vi "Electrical_Data_IEEE1459.vi"(6 "Config":cluster{"k":i32, "f":i32, "fs":i32}, 7 "fase a":cluster{"va(t)":dbl[], "ia(t)":dbl[]}, 8 "fase c":cluster{"vc(t)":dbl[], "ic(t)":dbl[]}, 11 "fase b":cluster{"vb(t)":dbl[], "ib(t)":dbl[]}) -> (0 "FASE C":T2, 3 "FASE B":T3, 4 "TRIFASICO":T1, 5 "FASE A":T4)   [LabVIEW 2017]
uses:
  <vilib>/Analysis/2dsp.llb/Real FFT.vi
  <vilib>/Analysis/baseanly.llb/Mean (DBL).vi
  <vilib>/Analysis/NI_AALPro.lvlib
  <vilib>/Analysis/NI_AALBase.lvlib
panel:
  in  "Cfg3F":T1
  in  "CfgC":T2
  in  "CfgB":T3
  in  "CfgA":T4
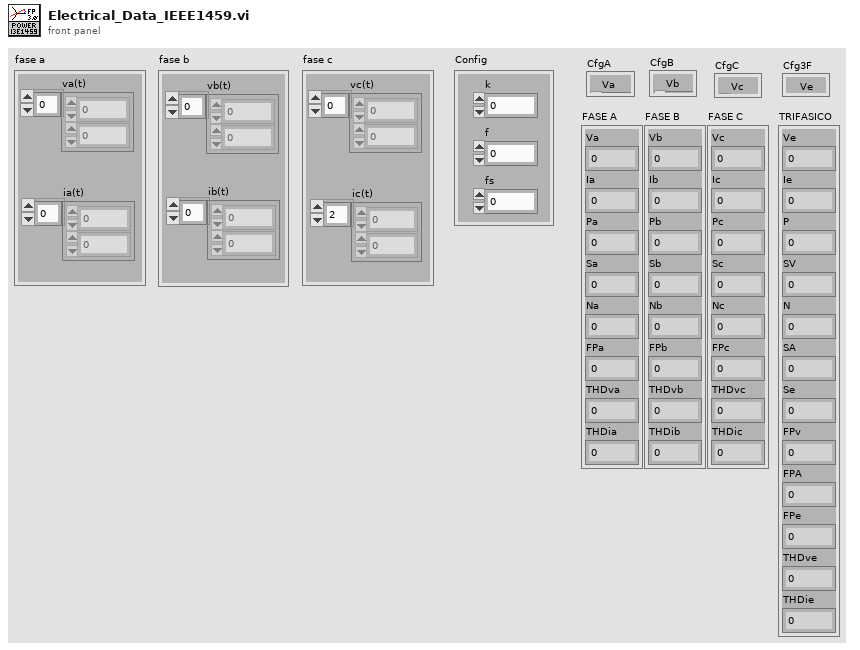
[diagram p1: front panel]
types:
  T1 = cluster{"Ve":dbl, "Ie":dbl, "P":dbl, "SV":dbl, "N":dbl, "SA":dbl, "Se":dbl, "FPv":dbl, "FPA":dbl, "FPe":dbl, "THDve":dbl, "THDie":dbl}
  T2 = cluster{"Vc":dbl, "Ic":dbl, "Pc":dbl, "Sc":dbl, "Nc":dbl, "FPc":dbl, "THDvc":dbl, "THDic":dbl}
  T3 = cluster{"Vb":dbl, "Ib":dbl, "Pb":dbl, "Sb":dbl, "Nb":dbl, "FPb":dbl, "THDvb":dbl, "THDib":dbl}
  T4 = cluster{"Va":dbl, "Ia":dbl, "Pa":dbl, "Sa":dbl, "Na":dbl, "FPa":dbl, "THDva":dbl, "THDia":dbl}
  T5 = cluster{cdb[], cdb[], cdb[], cdb[], cdb[], cdb[], cdb[], cdb[], cdb[], cdb[]}
  T6 = cluster{cdb[], cdb[], cdb[], cdb[], cdb[], cdb[]}
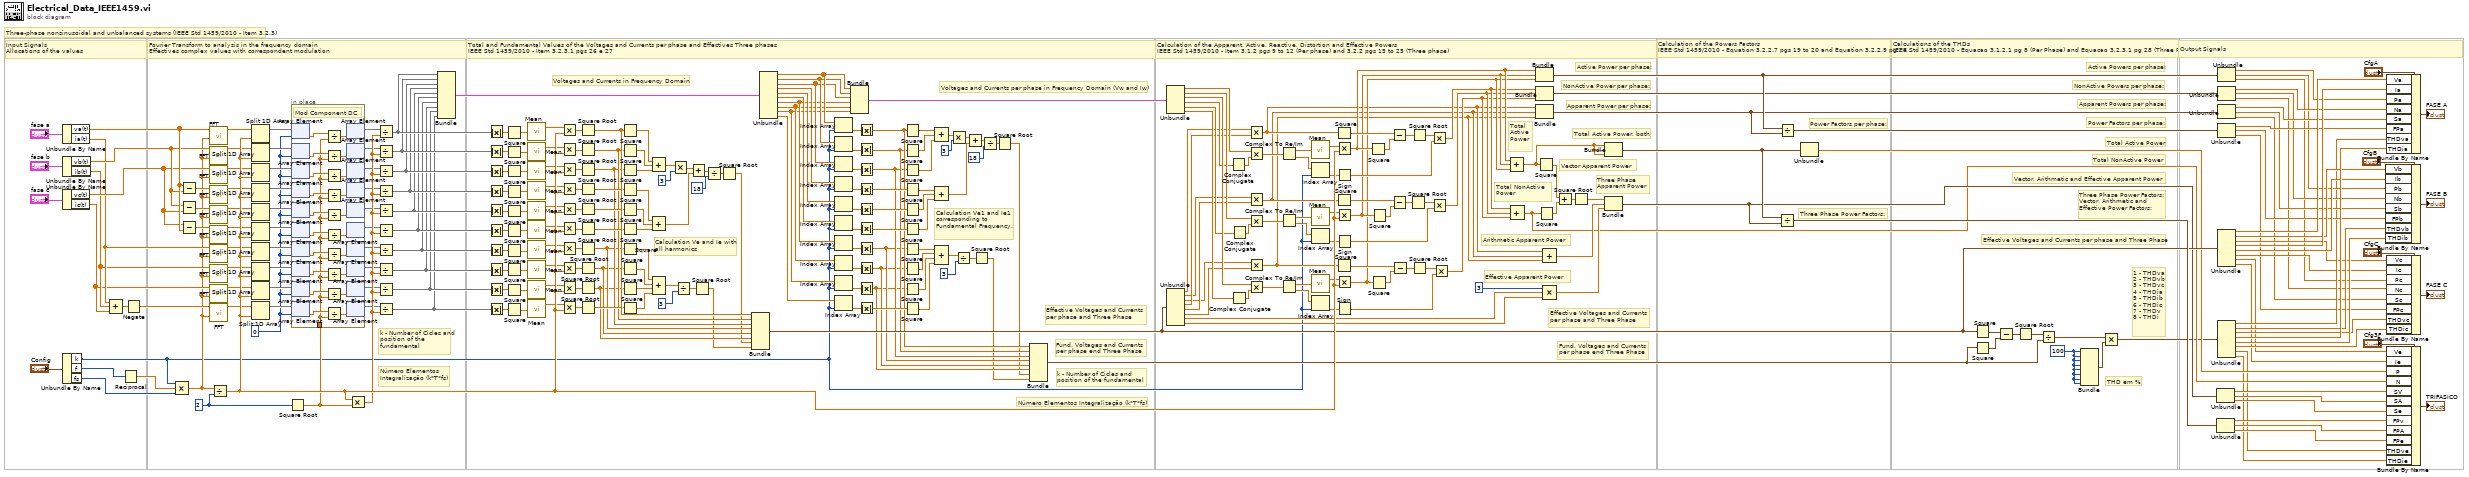
[diagram p0: block diagram]
diagram:
  w2 = i8 100
  w247 = 0 ("index")
  w268 = i8 2 ("y")
  # "THD em %"
  # "Three Phase Power Factors:"
  # "Power Factors per phase:"
  # "Vector, Arithmetic and Effective Apparent Power"
  # "Total Active Power"
  # "Active Powers per phase:"
  # "NonActive Powers per phase:"
  # "Apparent Powers per phase:"
  # "Total NonActive Power"
  # "Power Factors per phase:"
  # "Three Phase Power Factors:\nVector, Arithmetic and Effective Power Factors:"
  # "Effective Voltages and Currents per phase and Three Phase"
  # "1 - THDva\n2 - THDvb\n3 - THDvc\n4 - THDia\n5 - THDib\n6 - THDic\n7 - THDv\n8 - THDi"
  # "Three Phase Apparent Power"
  # "Total Active Power, both"
  # "Apparent Power per phase:"
  # "NonActive Power per phase:"
  # "Active Power per phase:"
  # "Effective Voltages and Currents per phase and Three Phase"
  # "Fund. Voltages and Currents per phase end Three Phase"
  # "Vector Apparent Power"
  # "Total NonActive Power"
  # "Total Active Power"
  # "Effective Apparent Power"
  # "Arithmetic Apparent Power"
  # "Voltages and Currents in Frequency Domain"
  # "Voltages and Currents per phase in Frequency Domain (Vw and Iw)"
  # "Fund. Voltages and Currents per phase end Three Phase"
  # "Effective Voltages and Currents per phase and Three Phase"
  # "Número Elementos Integralização (k*T*fs)"
  # "k - Number of Cicles and position of the fundamental"
  # "Calculation Ve1 and Ie1 corresponding to Fundamental Frequency."
  # "Calculation Ve and Ie with\nall harmonics"
  # "k - Number of Cicles and position of the fundamental"
  # "Número Elementos Integralização (k*T*fs)"
  # "Three-phase nonsinusoidal and unbalanced systems (IEEE Std 1459/2010 - Ítem 3.2.3)"
  # "Input Signals\nAllocations of the values"
  # "Output Signals"
  # "Calculations of the THDs\nIEEE Std 1459/2010 - Equacao 3.1.2.1 pg 8 (Per Phase) and Equacao 3.2.3.1 pg 28 (Three Phase)"
  # "Calculation of the Powers Factors\nIEEE Std 1459/2010 - Equation 3.2.2.7 pgs 19 to 20 and Equation 3.2.2.9 pg 24"
  # "Calculation of the Apparent, Active, Reactive, Distortion and Effective Powers\nIEEE Std 1459/2010 - Ítem 3.1.2 pgs 9 to 12 (Per phase) and 3.2.2 pgs 15 to 25 (Three phase)"
  # "Total and Fundamental Values of the Voltages and Currents per phase and Effectives Three phases\nIEEE Std 1459/2010 - Ítem 3.2.3.1 pgs 26 e 27"
  # "Fourier Transform to analysis in the frequency domain\nEffectives complex values with correspondent modulation"
  n1 = Unbundle By Name("fase a") -> ("va(t)"=w305:dbl[], "ia(t)"=w300:dbl[])
  n2 = Unbundle By Name("fase b") -> ("vb(t)"=w304:dbl[], "ib(t)"=w299:dbl[])
  n3 = Unbundle By Name("fase c") -> ("vc(t)"=w303:dbl[], "ic(t)"=w298:dbl[])
  n4 = Unbundle By Name("Config") -> ("k"=w15:i32, "f"=w13:i32, "fs"=w14:i32)
  n5 = Compound Arithmetic op=ADD(w300, w299, w298) -> (w287:dbl[])
  n6 = Reciprocal(x=w13) -> (1/x=w302:dbl)
  n7 = Negate(x=w287) -> (-x=w301:dbl[])
  n8 = Compound Arithmetic op=MULTIPLY(w15, w302, w14) -> (w280:dbl)
  n9 = Subtract(x=w305, y=w304) -> (x-y=w283:dbl[])
  n10 = Subtract(x=w304, y=w303) -> (x-y=w282:dbl[])
  n11 = Subtract(x=w303, y=w305) -> (x-y=w281:dbl[])
  n12 = call-poly <vilib>:"FFT.vi"("FFT size"=w280, "X"=w305) -> ("FFT {X}"=w279:cdb[])  [unwired: 8 in, 1 out]
  n13 = call-poly <vilib>:"FFT.vi"("FFT size"=w280, "X"=w304) -> ("FFT {X}"=w277:cdb[])  [unwired: 8 in, 1 out]
  n14 = call-poly <vilib>:"FFT.vi"("FFT size"=w280, "X"=w303) -> ("FFT {X}"=w276:cdb[])  [unwired: 8 in, 1 out]
  n15 = call-poly <vilib>:"FFT.vi"("FFT size"=w280, "X"=w283) -> ("FFT {X}"=w275:cdb[])  [unwired: 8 in, 1 out]
  n16 = call-poly <vilib>:"FFT.vi"("FFT size"=w280, "X"=w282) -> ("FFT {X}"=w274:cdb[])  [unwired: 8 in, 1 out]
  n17 = call-poly <vilib>:"FFT.vi"("FFT size"=w280, "X"=w281) -> ("FFT {X}"=w273:cdb[])  [unwired: 8 in, 1 out]
  n18 = call-poly <vilib>:"FFT.vi"("FFT size"=w280, "X"=w300) -> ("FFT {X}"=w272:cdb[])  [unwired: 8 in, 1 out]
  n19 = call-poly <vilib>:"FFT.vi"("FFT size"=w280, "X"=w299) -> ("FFT {X}"=w271:cdb[])  [unwired: 8 in, 1 out]
  n20 = call-poly <vilib>:"FFT.vi"("FFT size"=w280, "X"=w298) -> ("FFT {X}"=w270:cdb[])  [unwired: 8 in, 1 out]
  n21 = call-poly <vilib>:"FFT.vi"("FFT size"=w280, "X"=w301) -> ("FFT {X}"=w278:cdb[])  [unwired: 8 in, 1 out]
  n22 = Divide(x=w280, y=w268) -> (x/y=w306:dbl)
  n23 = Split 1D Array(array=w279, index=w306) -> (first subarray=w267:cdb[])  [unwired: 1 out]
  n24 = Split 1D Array(array=w277, index=w306) -> (first subarray=w266:cdb[])  [unwired: 1 out]
  n25 = Split 1D Array(array=w276, index=w306) -> (first subarray=w265:cdb[])  [unwired: 1 out]
  n26 = Split 1D Array(array=w275, index=w306) -> (first subarray=w264:cdb[])  [unwired: 1 out]
  n27 = Split 1D Array(array=w274, index=w306) -> (first subarray=w263:cdb[])  [unwired: 1 out]
  n28 = Split 1D Array(array=w273, index=w306) -> (first subarray=w262:cdb[])  [unwired: 1 out]
  n29 = Split 1D Array(array=w272, index=w306) -> (first subarray=w261:cdb[])  [unwired: 1 out]
  n30 = Split 1D Array(array=w271, index=w306) -> (first subarray=w260:cdb[])  [unwired: 1 out]
  n31 = Split 1D Array(array=w270, index=w306) -> (first subarray=w259:cdb[])  [unwired: 1 out]
  n32 = Split 1D Array(array=w278, index=w306) -> (first subarray=w258:cdb[])  [unwired: 1 out]
  n33 = Square Root(x=w268) -> (sqrt(x)=w246:dbl)
  n34 = in-place {
    in-place-border: w246 -> [w317]
    # "Mod Component DC"
    n35 = in-place-array #1(w267, w247) -> (w318:cdb)
    n36 = in-place-array #2(w266, w247) -> (w319:cdb)
    n37 = in-place-array #3(w265, w247) -> (w320:cdb)
    n38 = in-place-array #4(w264, w247) -> (w321:cdb)
    n39 = in-place-array #5(w263, w247) -> (w322:cdb)
    n40 = in-place-array #6(w262, w247) -> (w323:cdb)
    n41 = in-place-array #7(w261, w247) -> (w324:cdb)
    n42 = in-place-array #8(w260, w247) -> (w325:cdb)
    n43 = in-place-array #9(w259, w247) -> (w326:cdb)
    n44 = in-place-array #10(w258, w247) -> (w327:cdb)
    n45 = Divide(x=w318, y=w317) -> (x/y=w336:cdb)
    n46 = Divide(x=w319, y=w317) -> (x/y=w328:cdb)
    n47 = Divide(x=w320, y=w317) -> (x/y=w329:cdb)
    n48 = Divide(x=w321, y=w317) -> (x/y=w330:cdb)
    n49 = Divide(x=w322, y=w317) -> (x/y=w331:cdb)
    n50 = Divide(x=w323, y=w317) -> (x/y=w332:cdb)
    n51 = Divide(x=w324, y=w317) -> (x/y=w333:cdb)
    n52 = Divide(x=w325, y=w317) -> (x/y=w334:cdb)
    n53 = Divide(x=w326, y=w317) -> (x/y=w335:cdb)
    n54 = Divide(x=w327, y=w317) -> (x/y=w337:cdb)
    n55 = in-place-array #1(w336) -> (w255:cdb[])  [unwired: 1 out]
    n56 = in-place-array #2(w328) -> (w256:cdb[])  [unwired: 1 out]
    n57 = in-place-array #3(w329) -> (w257:cdb[])  [unwired: 1 out]
    n58 = in-place-array #4(w330) -> (w254:cdb[])  [unwired: 1 out]
    n59 = in-place-array #5(w331) -> (w253:cdb[])  [unwired: 1 out]
    n60 = in-place-array #6(w332) -> (w252:cdb[])  [unwired: 1 out]
    n61 = in-place-array #7(w333) -> (w251:cdb[])  [unwired: 1 out]
    n62 = in-place-array #8(w334) -> (w250:cdb[])  [unwired: 1 out]
    n63 = in-place-array #9(w335) -> (w249:cdb[])  [unwired: 1 out]
    n64 = in-place-array #10(w337) -> (w248:cdb[])  [unwired: 1 out]
  }
  n65 = Multiply(x=w306, y=w246) -> (x*y=w269:dbl)
  n66 = Divide(x=w255, y=w269) -> (x/y=w316:cdb[])
  n67 = Divide(x=w256, y=w269) -> (x/y=w315:cdb[])
  n68 = Divide(x=w257, y=w269) -> (x/y=w314:cdb[])
  n69 = Divide(x=w254, y=w269) -> (x/y=w313:cdb[])
  n70 = Divide(x=w253, y=w269) -> (x/y=w312:cdb[])
  n71 = Divide(x=w252, y=w269) -> (x/y=w311:cdb[])
  n72 = Divide(x=w251, y=w269) -> (x/y=w310:cdb[])
  n73 = Divide(x=w250, y=w269) -> (x/y=w309:cdb[])
  n74 = Divide(x=w249, y=w269) -> (x/y=w308:cdb[])
  n75 = Divide(x=w248, y=w269) -> (x/y=w307:cdb[])
  n76 = Bundle(w316, w315, w314, w313, w312, w311, w310, w309, w308, w307) -> (w297:T5)  [unwired: 1 in]
  n77 = Absolute Value(x=w316) -> (abs(x)=w245:dbl[])
  n78 = Absolute Value(x=w315) -> (abs(x)=w244:dbl[])
  n79 = Absolute Value(x=w314) -> (abs(x)=w243:dbl[])
  n80 = Absolute Value(x=w313) -> (abs(x)=w168:dbl[])
  n81 = Absolute Value(x=w312) -> (abs(x)=w242:dbl[])
  n82 = Absolute Value(x=w311) -> (abs(x)=w241:dbl[])
  n83 = Absolute Value(x=w310) -> (abs(x)=w240:dbl[])
  n84 = Absolute Value(x=w309) -> (abs(x)=w239:dbl[])
  n85 = Absolute Value(x=w308) -> (abs(x)=w238:dbl[])
  n86 = Absolute Value(x=w307) -> (abs(x)=w237:dbl[])
  n87 = Square(x=w245) -> (x^2=w227:dbl[])
  n88 = Square(x=w244) -> (x^2=w228:dbl[])
  n89 = Square(x=w243) -> (x^2=w229:dbl[])
  n90 = Square(x=w168) -> (x^2=w230:dbl[])
  n91 = Square(x=w242) -> (x^2=w231:dbl[])
  n92 = Square(x=w241) -> (x^2=w232:dbl[])
  n93 = Square(x=w240) -> (x^2=w233:dbl[])
  n94 = Square(x=w239) -> (x^2=w234:dbl[])
  n95 = Square(x=w238) -> (x^2=w235:dbl[])
  n96 = Square(x=w237) -> (x^2=w236:dbl[])
  n97 = call-poly <vilib>:"Mean.vi"("X"=w227) -> ("mean"=w226:dbl)  [unwired: 1 out]
  n98 = call-poly <vilib>:"Mean.vi"("X"=w228) -> ("mean"=w207:dbl)  [unwired: 1 out]
  n99 = call-poly <vilib>:"Mean.vi"("X"=w229) -> ("mean"=w208:dbl)  [unwired: 1 out]
  n100 = call-poly <vilib>:"Mean.vi"("X"=w230) -> ("mean"=w209:dbl)  [unwired: 1 out]
  n101 = call-poly <vilib>:"Mean.vi"("X"=w231) -> ("mean"=w210:dbl)  [unwired: 1 out]
  n102 = call-poly <vilib>:"Mean.vi"("X"=w232) -> ("mean"=w211:dbl)  [unwired: 1 out]
  n103 = call-poly <vilib>:"Mean.vi"("X"=w233) -> ("mean"=w212:dbl)  [unwired: 1 out]
  n104 = call-poly <vilib>:"Mean.vi"("X"=w234) -> ("mean"=w213:dbl)  [unwired: 1 out]
  n105 = call-poly <vilib>:"Mean.vi"("X"=w235) -> ("mean"=w214:dbl)  [unwired: 1 out]
  n106 = call-poly <vilib>:"Mean.vi"("X"=w236) -> ("mean"=w224:dbl)  [unwired: 1 out]
  n107 = Multiply(x=w226, y=w306) -> (x*y=w225:dbl)
  n108 = Multiply(x=w207, y=w306) -> (x*y=w222:dbl)
  n109 = Multiply(x=w208, y=w306) -> (x*y=w221:dbl)
  n110 = Multiply(x=w209, y=w306) -> (x*y=w220:dbl)
  n111 = Multiply(x=w210, y=w306) -> (x*y=w219:dbl)
  n112 = Multiply(x=w211, y=w306) -> (x*y=w218:dbl)
  n113 = Multiply(x=w212, y=w306) -> (x*y=w217:dbl)
  n114 = Multiply(x=w213, y=w306) -> (x*y=w216:dbl)
  n115 = Multiply(x=w214, y=w306) -> (x*y=w215:dbl)
  n116 = Multiply(x=w224, y=w306) -> (x*y=w223:dbl)
  n117 = Square Root(x=w225) -> (sqrt(x)=w147:dbl)
  n118 = Square Root(x=w222) -> (sqrt(x)=w128:dbl)
  n119 = Square Root(x=w221) -> (sqrt(x)=w127:dbl)
  n120 = Square Root(x=w220) -> (sqrt(x)=w146:dbl)
  n121 = Square Root(x=w219) -> (sqrt(x)=w145:dbl)
  n122 = Square Root(x=w218) -> (sqrt(x)=w144:dbl)
  n123 = Square Root(x=w217) -> (sqrt(x)=w126:dbl)
  n124 = Square Root(x=w216) -> (sqrt(x)=w125:dbl)
  n125 = Square Root(x=w215) -> (sqrt(x)=w124:dbl)
  n126 = Square Root(x=w223) -> (sqrt(x)=w143:dbl)
  n127 = Square(x=w147) -> (x^2=w200:dbl)
  n128 = Square(x=w128) -> (x^2=w199:dbl)
  n129 = Square(x=w127) -> (x^2=w198:dbl)
  n130 = Square(x=w146) -> (x^2=w197:dbl)
  n131 = Square(x=w145) -> (x^2=w196:dbl)
  n132 = Square(x=w144) -> (x^2=w195:dbl)
  n133 = Square(x=w126) -> (x^2=w205:dbl)
  n134 = Square(x=w125) -> (x^2=w204:dbl)
  n135 = Square(x=w124) -> (x^2=w203:dbl)
  n136 = Square(x=w143) -> (x^2=w202:dbl)
  n137 = Compound Arithmetic op=ADD(w200, w199, w198) -> (w194:dbl)
  n138 = Compound Arithmetic op=ADD(w197, w196, w195) -> (w192:dbl)
  n139 = Compound Arithmetic op=ADD(w205, w204, w203, w202) -> (w201:dbl)
  n140 = Multiply(x=w194, y=i8 3) -> (x*y=w193:dbl)
  n141 = Divide(x=w201, y=i8 3) -> (x/y=w206:dbl)
  n142 = Add(x=w193, y=w192) -> (x+y=w190:dbl)
  n143 = Square Root(x=w206) -> (sqrt(x)=w123:dbl)
  n144 = Divide(x=w190, y=i8 18) -> (x/y=w191:dbl)
  n145 = Square Root(x=w191) -> (sqrt(x)=w122:dbl)
  n146 = Bundle(w147, w128, w127, w126, w125, w124, w122, w123) -> (w288:cluster{dbl, dbl, dbl, dbl, dbl, dbl, dbl, dbl})  [unwired: 1 in]
  n147 = Unbundle(w297) -> (w134:cdb[], w133:cdb[], w132:cdb[], w151:cdb[], w150:cdb[], w149:cdb[], w131:cdb[], w130:cdb[], w129:cdb[], w148:cdb[])
  n148 = Index Array(array=w134, index=w15) -> (element=w154:cdb)
  n149 = Index Array(array=w133, index=w15) -> (element=w155:cdb)
  n150 = Index Array(array=w132, index=w15) -> (element=w156:cdb)
  n151 = Index Array(array=w151, index=w15) -> (element=w157:cdb)
  n152 = Index Array(array=w150, index=w15) -> (element=w160:cdb)
  n153 = Index Array(array=w149, index=w15) -> (element=w161:cdb)
  n154 = Index Array(array=w131, index=w15) -> (element=w163:cdb)
  n155 = Index Array(array=w130, index=w15) -> (element=w164:cdb)
  n156 = Index Array(array=w129, index=w15) -> (element=w165:cdb)
  n157 = Index Array(array=w148, index=w15) -> (element=w166:cdb)
  n158 = Bundle(w134, w133, w132, w131, w130, w129) -> (w296:T6)  [unwired: 1 in]
  n159 = Absolute Value(x=w154) -> (abs(x)=w142:dbl)
  n160 = Absolute Value(x=w155) -> (abs(x)=w141:dbl)
  n161 = Absolute Value(x=w156) -> (abs(x)=w140:dbl)
  n162 = Absolute Value(x=w157) -> (abs(x)=w158:dbl)
  n163 = Absolute Value(x=w160) -> (abs(x)=w159:dbl)
  n164 = Absolute Value(x=w161) -> (abs(x)=w162:dbl)
  n165 = Absolute Value(x=w163) -> (abs(x)=w139:dbl)
  n166 = Absolute Value(x=w164) -> (abs(x)=w138:dbl)
  n167 = Absolute Value(x=w165) -> (abs(x)=w137:dbl)
  n168 = Absolute Value(x=w166) -> (abs(x)=w167:dbl)
  n169 = Square(x=w142) -> (x^2=w174:dbl)
  n170 = Square(x=w141) -> (x^2=w175:dbl)
  n171 = Square(x=w140) -> (x^2=w153:dbl)
  n172 = Square(x=w158) -> (x^2=w176:dbl)
  n173 = Square(x=w159) -> (x^2=w177:dbl)
  n174 = Square(x=w162) -> (x^2=w178:dbl)
  n175 = Square(x=w139) -> (x^2=w170:dbl)
  n176 = Square(x=w138) -> (x^2=w171:dbl)
  n177 = Square(x=w137) -> (x^2=w152:dbl)
  n178 = Square(x=w167) -> (x^2=w172:dbl)
  n179 = Compound Arithmetic op=ADD(w174, w175, w153) -> (w179:dbl)
  n180 = Compound Arithmetic op=ADD(w176, w177, w178) -> (w181:dbl)
  n181 = Compound Arithmetic op=ADD(w170, w171, w152, w172) -> (w173:dbl)
  n182 = Multiply(x=w179, y=i8 3) -> (x*y=w180:dbl)
  n183 = Divide(x=w173, y=i8 3) -> (x/y=w169:dbl)
  n184 = Add(x=w180, y=w181) -> (x+y=w183:dbl)
  n185 = Square Root(x=w169) -> (sqrt(x)=w135:dbl)
  n186 = Divide(x=w183, y=i8 18) -> (x/y=w182:dbl)
  n187 = Square Root(x=w182) -> (sqrt(x)=w136:dbl)
  n188 = Bundle(w142, w141, w140, w139, w138, w137, w136, w135) -> (w294:cluster{dbl, dbl, dbl, dbl, dbl, dbl, dbl, dbl})  [unwired: 1 in]
  n189 = Unbundle(w296) -> (w84:cdb[], w83:cdb[], w82:cdb[], w81:cdb[], w80:cdb[], w79:cdb[])
  n190 = Unbundle(w288) -> (w59:dbl, w57:dbl, w55:dbl, w58:dbl, w56:dbl, w54:dbl, w78:dbl, w77:dbl)
  n191 = Complex Conjugate(1:w81) -> (0:w119:cdb[])
  n192 = Complex Conjugate(1:w79) -> (0:w121:cdb[])
  n193 = Complex Conjugate(1:w80) -> (0:w120:cdb[])
  n194 = Multiply(x=w59, y=w58) -> (x*y=w70:dbl)
  n195 = Multiply(x=w84, y=w119) -> (x*y=w118:cdb[])
  n196 = Multiply(x=w57, y=w56) -> (x*y=w69:dbl)
  n197 = Multiply(x=w83, y=w120) -> (x*y=w117:cdb[])
  n198 = Multiply(x=w55, y=w54) -> (x*y=w68:dbl)
  n199 = Multiply(x=w82, y=w121) -> (x*y=w116:cdb[])
  n200 = Complex To Re/Im(x + iy=w118) -> (x=w115:dbl[], y=w105:dbl[])
  n201 = Complex To Re/Im(x + iy=w117) -> (x=w114:dbl[], y=w104:dbl[])
  n202 = Complex To Re/Im(x + iy=w116) -> (x=w113:dbl[], y=w103:dbl[])
  n203 = call-poly <vilib>:"Mean.vi"("X"=w115) -> ("mean"=w112:dbl)  [unwired: 1 out]
  n204 = Index Array(array=w105, index=w15) -> (element=w95:dbl)
  n205 = call-poly <vilib>:"Mean.vi"("X"=w114) -> ("mean"=w110:dbl)  [unwired: 1 out]
  n206 = Index Array(array=w104, index=w15) -> (element=w96:dbl)
  n207 = call-poly <vilib>:"Mean.vi"("X"=w113) -> ("mean"=w111:dbl)  [unwired: 1 out]
  n208 = Index Array(array=w103, index=w15) -> (element=w97:dbl)
  n209 = Square(x=w70) -> (x^2=w101:dbl)
  n210 = Square(x=w69) -> (x^2=w98:dbl)
  n211 = Square(x=w68) -> (x^2=w91:dbl)
  n212 = Multiply(x=w112, y=w306) -> (x*y=w76:dbl)
  n213 = Sign(1:w95) -> (0:w94:dbl)
  n214 = Multiply(x=w110, y=w306) -> (x*y=w75:dbl)
  n215 = Sign(1:w96) -> (0:w93:dbl)
  n216 = Multiply(x=w111, y=w306) -> (x*y=w74:dbl)
  n217 = Sign(1:w97) -> (0:w92:dbl)
  n218 = Square(x=w76) -> (x^2=w102:dbl)
  n219 = Square(x=w74) -> (x^2=w99:dbl)
  n220 = Square(x=w75) -> (x^2=w100:dbl)
  n221 = Subtract(x=w101, y=w102) -> (x-y=w90:dbl)
  n222 = Subtract(x=w98, y=w100) -> (x-y=w88:dbl)
  n223 = Subtract(x=w91, y=w99) -> (x-y=w86:dbl)
  n224 = Square Root(x=w88) -> (sqrt(x)=w87:dbl)
  n225 = Square Root(x=w90) -> (sqrt(x)=w89:dbl)
  n226 = Square Root(x=w86) -> (sqrt(x)=w85:dbl)
  n227 = Multiply(x=w89, y=w94) -> (x*y=w73:dbl)
  n228 = Multiply(x=w87, y=w93) -> (x*y=w72:dbl)
  n229 = Multiply(x=w85, y=w92) -> (x*y=w71:dbl)
  n230 = Compound Arithmetic op=ADD(w76, w75, w74) -> (w64:dbl)
  n231 = Compound Arithmetic op=ADD(w73, w72, w71) -> (w23:dbl)
  n232 = Bundle(w76, w75, w74) -> (w293:cluster{dbl, dbl, dbl})  [unwired: 1 in]
  n233 = Bundle(w73, w72, w71) -> (w292:cluster{dbl, dbl, dbl})  [unwired: 1 in]
  n234 = Bundle(w70, w69, w68) -> (w291:cluster{dbl, dbl, dbl})  [unwired: 1 in]
  n235 = Square(x=w64) -> (x^2=w107:dbl)
  n236 = Square(x=w23) -> (x^2=w106:dbl)
  n237 = Compound Arithmetic op=ADD(w70, w69, w68) -> (w66:dbl)
  n238 = Compound Arithmetic op=MULTIPLY(i8 3 ("value"), w78, w77) -> (w67:dbl)
  n239 = Add(x=w107, y=w106) -> (x+y=w108:dbl)
  n240 = Square Root(x=w108) -> (sqrt(x)=w65:dbl)
  n241 = Bundle(w65, w66, w67) -> (w25:cluster{dbl, dbl, dbl})  [unwired: 1 in]
  n242 = Bundle(w64, w64, w64) -> (w295:cluster{dbl, dbl, dbl})  [unwired: 1 in]
  n243 = Divide(x=w295, y=w25) -> (x/y=w289:cluster{dbl, dbl, dbl})
  n244 = Divide(x=w293, y=w291) -> (x/y=w290:cluster{dbl, dbl, dbl})
  n245 = Unbundle(w295) -> (w24:dbl)  [unwired: 2 out]
  n246 = Square(x=w288) -> (x^2=w63:cluster{dbl, dbl, dbl, dbl, dbl, dbl, dbl, dbl})
  n247 = Square(x=w294) -> (x^2=w62:cluster{dbl, dbl, dbl, dbl, dbl, dbl, dbl, dbl})
  n248 = Subtract(x=w63, y=w62) -> (x-y=w60:cluster{dbl, dbl, dbl, dbl, dbl, dbl, dbl, dbl})
  n249 = Square Root(x=w60) -> (sqrt(x)=w61:cluster{dbl, dbl, dbl, dbl, dbl, dbl, dbl, dbl})
  n250 = Divide(x=w61, y=w294) -> (x/y=w4:cluster{dbl, dbl, dbl, dbl, dbl, dbl, dbl, dbl})
  n251 = Bundle(w2, w2, w2, w2, w2, w2, w2, w2) -> (w1:cluster{i8, i8, i8, i8, i8, i8, i8, i8})  [unwired: 1 in]
  n252 = Multiply(x=w4, y=w1) -> (x*y=w3:cluster{dbl, dbl, dbl, dbl, dbl, dbl, dbl, dbl})
  n253 = Unbundle(w25) -> (w22:dbl, w21:dbl, w20:dbl)
  n254 = Unbundle(w289) -> (w19:dbl, w18:dbl, w17:dbl)
  n255 = Unbundle(w293) -> (w50:dbl, w42:dbl, w32:dbl)
  n256 = Unbundle(w292) -> (w49:dbl, w41:dbl, w31:dbl)
  n257 = Unbundle(w291) -> (w48:dbl, w40:dbl, w30:dbl)
  n258 = Unbundle(w290) -> (w46:dbl, w39:dbl, w29:dbl)
  n259 = Unbundle(w288) -> (w52:dbl, w44:dbl, w34:dbl, w51:dbl, w43:dbl, w33:dbl, w12:dbl, w11:dbl)
  n260 = Unbundle(w3) -> (w36:dbl, w38:dbl, w28:dbl, w47:dbl, w37:dbl, w26:dbl, w10:dbl, w9:dbl)
  n261 = Bundle By Name(cluster="CfgB", "Vb"=w44, "Ib"=w43, "Pb"=w42, "Nb"=w41, "Sb"=w40, "FPb"=w39, "THDvb"=w38, "THDib"=w37) -> (→"FASE B":T3)
  n262 = Bundle By Name(cluster="CfgA", "Va"=w52, "Ia"=w51, "Pa"=w50, "Na"=w49, "Sa"=w48, "FPa"=w46, "THDva"=w36, "THDia"=w47) -> (→"FASE A":T4)
  n263 = Bundle By Name(cluster="CfgC", "Vc"=w34, "Ic"=w33, "Pc"=w32, "Nc"=w31, "Sc"=w30, "FPc"=w29, "THDvc"=w28, "THDic"=w26) -> (→"FASE C":T2)
  n264 = Bundle By Name(cluster="Cfg3F", "Ve"=w12, "Ie"=w11, "P"=w24, "N"=w23, "SV"=w22, "SA"=w21, "Se"=w20, "FPv"=w19, "FPA"=w18, "FPe"=w17, "THDve"=w10, "THDie"=w9) -> (→"TRIFASICO":T1)
